vi "set_query infusion volume.vi"(0 "VISA resource name":refnum<visa-resource-name>, 5 "Query?":bool, 7 "Volume Units (0:ml)":u16(ring) items=["microliters", "nanoliters", "milliliters"], 9 "Volume":i32=1 min=0 max=999 step=1, 11 "error in (no error)":errorcluster) -> (4 "VISA resource name out":refnum<visa-resource-name>, 6 "Output infusion volume":string, 15 "error out":errorcluster)   [LabVIEW 2016]
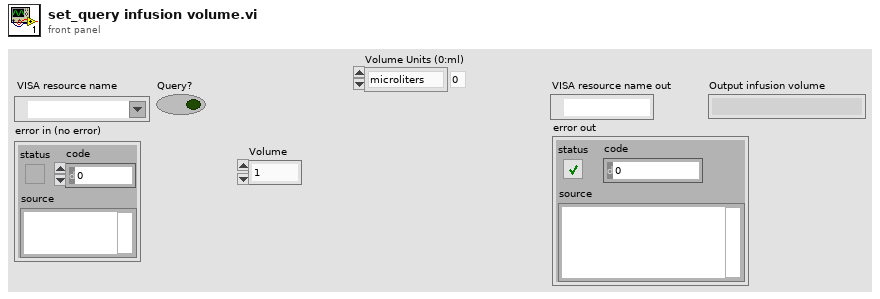
[diagram p1: front panel]
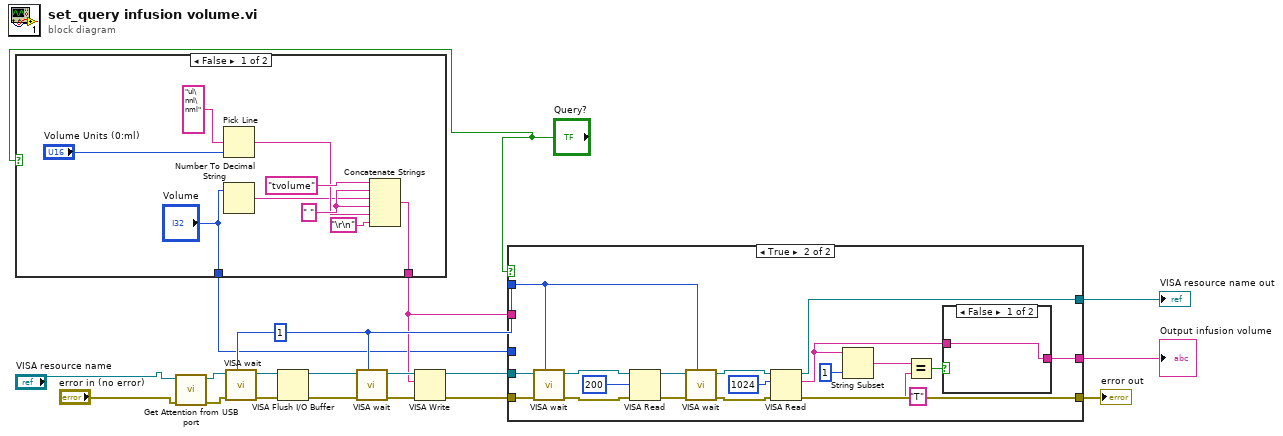
[diagram p0: block diagram]
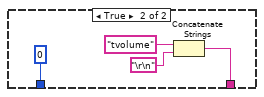
[diagram p2: hidden frame]
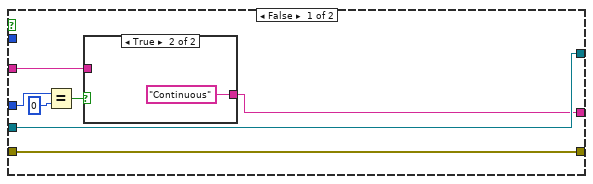
[diagram p3: hidden frame]
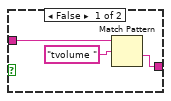
[diagram p4: hidden frame]
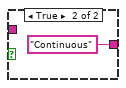
[diagram p5: hidden frame]
diagram:
  w9 = u32 1 ("milliseconds to wait")
  n1 = case shown="False" "Query?" {
    tunnel: [w21 w29] -> w7
    tunnel: ["Volume" 0 ("Volume")] -> w6
    frame False {
      w25 = " " ("string")
      n2 = Pick Line(multi-line string="ul\nnl\nml", line index="Volume Units (0:ml)") -> (output string=w24:string)  [unwired: 1 in]
      n3 = Number To Decimal String(number="Volume") -> (decimal integer string=w22:string)  [unwired: 1 in]
      n4 = Concatenate Strings("tvolume" ("string"), w25, w22, w25, w24, "\r\n") -> (w21:string)
    }
    frame True {
      n5 = Concatenate Strings("tvolume" ("string"), "\r\n") -> (w29:string)
    }
  }
  n6 = call "Get Attention from USB port.vi"("error in (no error)"="error in (no error)", "VISA resource name"="VISA resource name") -> ("error out"=w3:errorcluster, "VISA resource name out"=w4:refnum<visa-resource-name>)  [unwired: 8 in]
  n7 = call <userlib>:"VISA wait.vi"("VISA resource name"=w4, "error in (no error)"=w3, "milliseconds to wait"=w9) -> ("VISA resource name out"=w18:refnum<visa-resource-name>, "error out"=w19:errorcluster)  [unwired: 6 in]
  n8 = VISA Flush I/O Buffer(VISA resource name=w18, error in (no error)=w19) -> (VISA resource name out=w17:refnum<visa-resource-name>, error out=w16:errorcluster)  [unwired: 1 in]
  n9 = call <userlib>:"VISA wait.vi"("VISA resource name"=w17, "error in (no error)"=w16, "milliseconds to wait"=w9) -> ("VISA resource name out"=w14:refnum<visa-resource-name>, "error out"=w15:errorcluster)  [unwired: 6 in]
  n10 = VISA Write(VISA resource name=w14, write buffer=w7, error in (no error)=w15) -> (VISA resource name out=w13:refnum<visa-resource-name>, error out=w12:errorcluster)  [unwired: 1 out]
  n11 = case shown="True" "Query?" {
    tunnel: w13 -> [w39 w62]
    tunnel: w12 -> [w38 w61]
    tunnel: [w39 w54] -> w11
    tunnel: [w38 w53] -> w10
    tunnel: w9 -> [_ w52]
    tunnel: [w36 w46] -> w8
    tunnel: w7 -> [w37 _]
    tunnel: w6 -> [w35 _]
    frame False {
      n12 = Equal?(x=w35, y=0) -> (x = y?=w33:bool)
      n13 = case shown="True" w33 {
        tunnel: w37 -> [w42 _]
        tunnel: [w40 "Continuous"] -> w36
        frame False {
          n14 = Match Pattern(string=w42, regular expression="tvolume ") -> (after substring=w40:string)  [unwired: 1 in, 3 out]
        }
        frame True {
        }
      }
    }
    frame True {
      n15 = call <userlib>:"VISA wait.vi"("VISA resource name"=w62, "error in (no error)"=w61, "milliseconds to wait"=w52) -> ("VISA resource name out"=w59:refnum<visa-resource-name>, "error out"=w60:errorcluster)  [unwired: 6 in]
      n16 = VISA Read(VISA resource name=w59, byte count=u32 200, error in (no error)=w60) -> (VISA resource name out=w58:refnum<visa-resource-name>, error out=w57:errorcluster)  [unwired: 2 out]
      n17 = call <userlib>:"VISA wait.vi"("VISA resource name"=w58, "error in (no error)"=w57, "milliseconds to wait"=w52) -> ("VISA resource name out"=w55:refnum<visa-resource-name>, "error out"=w56:errorcluster)  [unwired: 6 in]
      n18 = VISA Read(VISA resource name=w55, byte count=u32 1024, error in (no error)=w56) -> (VISA resource name out=w54:refnum<visa-resource-name>, read buffer=w45:string, error out=w53:errorcluster)  [unwired: 1 out]
      n19 = String Subset(string=w45, length (rest)=1 ("length (rest)")) -> (substring=w49:string)  [unwired: 1 in]
      n20 = Equal?(x=w49, y="T") -> (x = y?=w47:bool)
      n21 = case shown="False" w47 {
        tunnel: [w63 "Continuous"] -> w46
        tunnel: w45 -> [w63 _]
        frame False {
        }
        frame True {
        }
      }
    }
  }
  "VISA resource name out" <- w11
  "error out" <- w10
  "Output infusion volume" <- w8
